vi "ChangeHeadDir.vi"(8 "error in (no error)":errorcluster, 10 "UnitDirection":T1, 11 "Snake in":refnum<class "Snake.lvclass">) -> (0 "error out":errorcluster, 3 "Snake out":refnum<class "Snake.lvclass">)   [LabVIEW 2018, in "Snake.lvclass"]
uses:
  Snake.lvclass
  Typedefs/UnitDirection.ctl
  Snake.lvclass/Snake.ctl
  BodyCell/SnakeBodyCell.lvclass
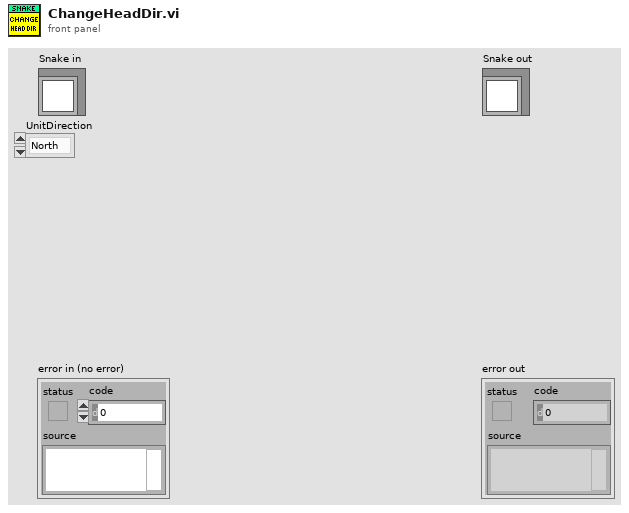
[diagram p1: front panel]
types:
  T1 = typedef "UnitDirection.ctl" = enum16{"North", "East", "South", "West"}
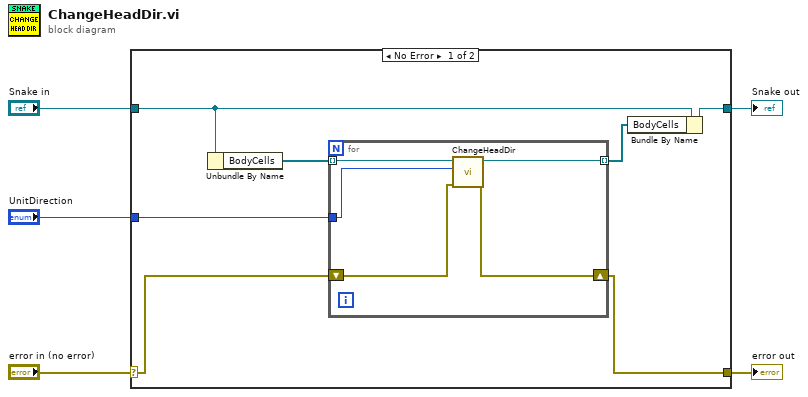
[diagram p0: block diagram]
diagram:
  n1 = case shown="No Error" "error in (no error)" {
    selector: "error in (no error)" -> [w8 w19]
    tunnel: [w7 w19] -> w4
    tunnel: [w10 w18] -> w2
    tunnel: "Snake in" -> [w11 w18]
    tunnel: "UnitDirection" -> [w6 _]
    frame No Error {
      n2 = Unbundle By Name(w11) -> ("BodyCells"=w12:refnum<class "SnakeBodyCell.lvclass">[])
      n3 = for {
        tunnel: [w16] -> w9 mode=indexing
        tunnel: w12 -> [w17] mode=indexing
        shift-right: [w14] -> w7
        shift-left: w8 -> [w15]
        tunnel: w6 -> [w13]
        n4 = call "ChangeHeadDir.vi"("error in (no error)"=w15, "UnitDirection"=w13, "SnakeBodyCell in"=w17) -> ("error out"=w14:errorcluster, "SnakeBodyCell out"=w16:refnum<class "SnakeBodyCell.lvclass">)  [unwired: 7 in]
      }
      n5 = Bundle By Name(cluster=w11, "BodyCells"=w9) -> (w10:refnum<class "Snake.lvclass">)
    }
    frame Error {
    }
  }
  "error out" <- w4
  "Snake out" <- w2
